vi "Set Pass Fail Leds.vi"(8 "error in":errorcluster, 9 "Fail Led":bool, 10 "Pass Led":bool, 11 "Task In":refnum<k21>) -> (0 "error out":errorcluster)   [LabVIEW 2018]
uses:
  <vilib>/DAQmx/write.llb/DAQmx Write (Digital 1D Bool 1Chan 1Samp).vi
  <vilib>/DAQmx/miscellaneous.llb/DAQmx Fill In Error Info.vi
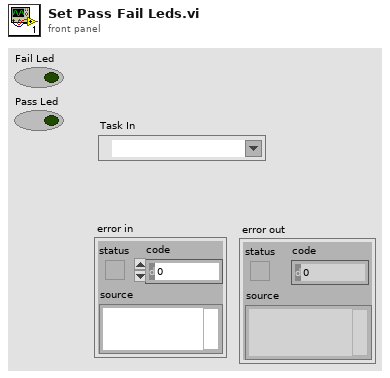
[diagram p1: front panel]
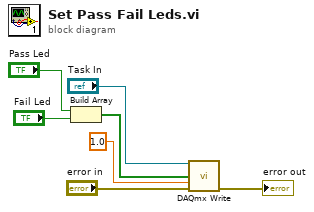
[diagram p0: block diagram]
diagram:
  n1 = Build Array("Pass Led", "Fail Led") -> (w3:bool[])
  n2 = call-poly <vilib>:"DAQmx Write.vi"("task/channels in"="Task In", "data"=w3, "timeout"=1.0, "error in"="error in") -> ("error out"=→"error out":errorcluster)  [unwired: 9 in, 2 out]
